vi "Draw Bot.vi"(7 "Angle":dbl, 9 "new picture in":picture, 10 "Robot Y":dbl, 11 "Robot X":dbl) -> (3 "new picture out":picture)   [LabVIEW 2013]
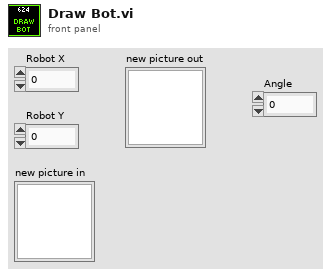
[diagram p1: front panel]
types:
  T1 = cluster{"left":i16, "top":i16, "right":i16, "bottom":i16}
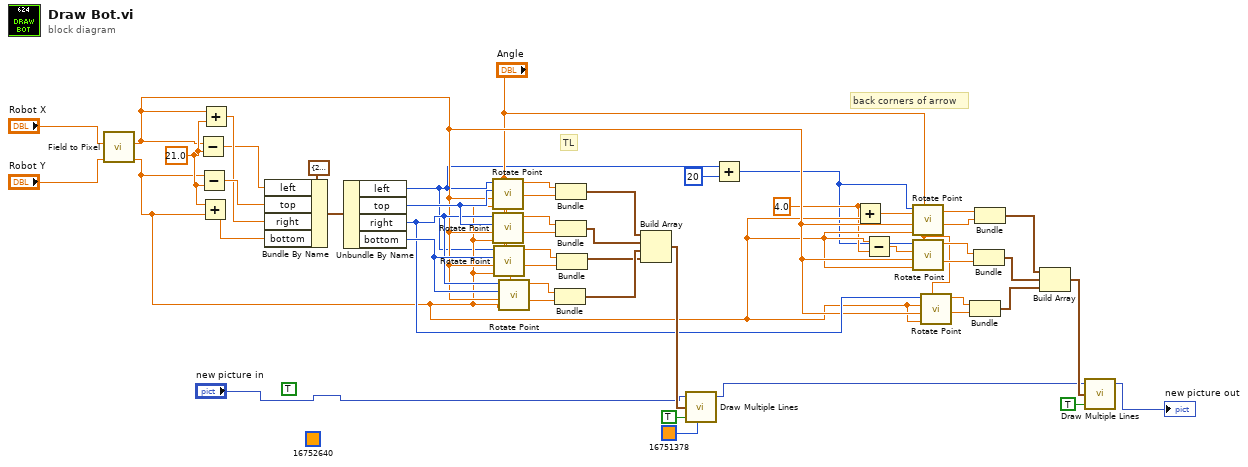
[diagram p0: block diagram]
diagram:
  w10 = 4.0
  w49 = 21.0 ("y")
  (unwired) TRUE ("fill?(F)")
  (unwired) u32 16752640 ("color(black)")
  # "back corners of arrow"
  # "TL"
  n1 = call "Field to Pixel.vi"("Field Coordinate Y"="Robot Y", "Field Coordinate X"="Robot X") -> ("Pixel Y"=w11:dbl, "Pixel X"=w13:dbl)  [unwired: 8 in]
  n2 = Subtract(x=w13, y=w49) -> (x-y=w43:dbl)
  n3 = Subtract(x=w11, y=w49) -> (x-y=w48:dbl)
  n4 = Add(x=w49, y=w11) -> (x+y=w50:dbl)
  n5 = Add(x=w13, y=w49) -> (x+y=w47:dbl)
  n6 = Bundle By Name(cluster=T1 {"left"=265, "top"=0, "right"=270, "bottom"=405} ("rect"), "left"=w43, "top"=w48, "right"=w47, "bottom"=w50) -> (w30:T1)
  n7 = Unbundle By Name(w30) -> ("left"=w3:i16, "top"=w42:i16, "right"=w23:i16, "bottom"=w41:i16)
  n8 = call "Rotate Point.vi"("Angle"="Angle", "Center Y"=w11, "Center X"=w13, "Y"=w42, "X"=w3) -> ("Y"=w39:dbl, "X"=w40:dbl)  [unwired: 5 in]
  n9 = call "Rotate Point.vi"("Angle"="Angle", "Center Y"=w11, "Center X"=w13, "Y"=w42, "X"=w23) -> ("Y"=w37:dbl, "X"=w38:dbl)  [unwired: 5 in]
  n10 = call "Rotate Point.vi"("Angle"="Angle", "Center Y"=w11, "Center X"=w13, "Y"=w41, "X"=w3) -> ("Y"=w35:dbl, "X"=w36:dbl)  [unwired: 5 in]
  n11 = call "Rotate Point.vi"("Angle"="Angle", "Center Y"=w11, "Center X"=w13, "Y"=w41, "X"=w23) -> ("Y"=w33:dbl, "X"=w34:dbl)  [unwired: 5 in]
  n12 = Bundle("X"=w34, "Y"=w33) -> (w26:cluster{"X":dbl, "Y":dbl})  [unwired: 1 in]
  n13 = Bundle("X"=w40, "Y"=w39) -> (w28:cluster{"X":dbl, "Y":dbl})  [unwired: 1 in]
  n14 = Bundle("X"=w38, "Y"=w37) -> (w27:cluster{"X":dbl, "Y":dbl})  [unwired: 1 in]
  n15 = Bundle("X"=w36, "Y"=w35) -> (w25:cluster{"X":dbl, "Y":dbl})  [unwired: 1 in]
  n16 = Build Array(w28, w27, w26, w25) -> (w32:cluster{"X":dbl, "Y":dbl}[])
  n17 = call <vilib>:"Draw Multiple Lines.vi"("picture"="new picture in", "line endpoints"=w32, "fill?(F)"=TRUE, "color(black)"=u32 16751378) -> ("new picture"=w15:picture)  [unwired: 5 in]
  n18 = Add(x=w3, y=i16 20) -> (x+y=w1:i16)
  n19 = Add(x=w10, y=w11) -> (x+y=w12:dbl)
  n20 = Subtract(x=w11, y=w10) -> (x-y=w9:dbl)
  n21 = call "Rotate Point.vi"("Angle"="Angle", "Center Y"=w11, "Center X"=w13, "Y"=w12, "X"=w1) -> ("Y"=w7:dbl, "X"=w8:dbl)  [unwired: 5 in]
  n22 = call "Rotate Point.vi"("Angle"="Angle", "Center Y"=w11, "Center X"=w13, "Y"=w9, "X"=w1) -> ("Y"=w21:dbl, "X"=w22:dbl)  [unwired: 5 in]
  n23 = call "Rotate Point.vi"("Angle"="Angle", "Center Y"=w11, "Center X"=w13, "Y"=w11, "X"=w23) -> ("Y"=w19:dbl, "X"=w20:dbl)  [unwired: 5 in]
  n24 = Bundle("X"=w20, "Y"=w19) -> (w17:cluster{"X":dbl, "Y":dbl})  [unwired: 1 in]
  n25 = Bundle("X"=w22, "Y"=w21) -> (w18:cluster{"X":dbl, "Y":dbl})  [unwired: 1 in]
  n26 = Bundle("X"=w8, "Y"=w7) -> (w5:cluster{"X":dbl, "Y":dbl})  [unwired: 1 in]
  n27 = Build Array(w5, w18, w17) -> (w16:cluster{"X":dbl, "Y":dbl}[])
  n28 = call <vilib>:"Draw Multiple Lines.vi"("picture"=w15, "line endpoints"=w16, "fill?(F)"=TRUE) -> ("new picture"=→"new picture out":picture)  [unwired: 6 in]
